vi "Create.vi"(8 "error in (no error)":errorcluster, 10 "Debug Data Cluster":T1) -> (0 "error out":errorcluster, 3 "Debug Data out":refnum<class "Debug Data.lvclass">)   [LabVIEW 2020, in "Debug Data.lvclass"]
uses:
  Debug Data.lvclass
  Raw Debug Data.ctl
  Debug Data.lvclass/Debug Data.ctl
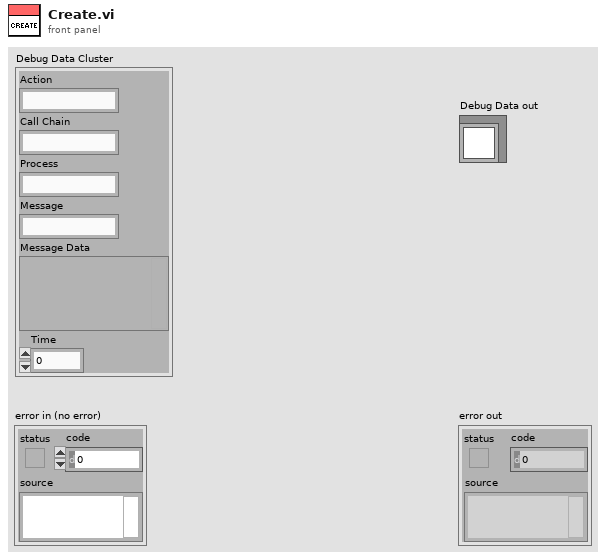
[diagram p1: front panel]
types:
  T1 = typedef "Debug Data.lvclass/Raw Debug Data.ctl" = cluster{"Action":string, "Call Chain":string, "Process":string, "Message":string, "Message Data":variant, "Time":dbl}
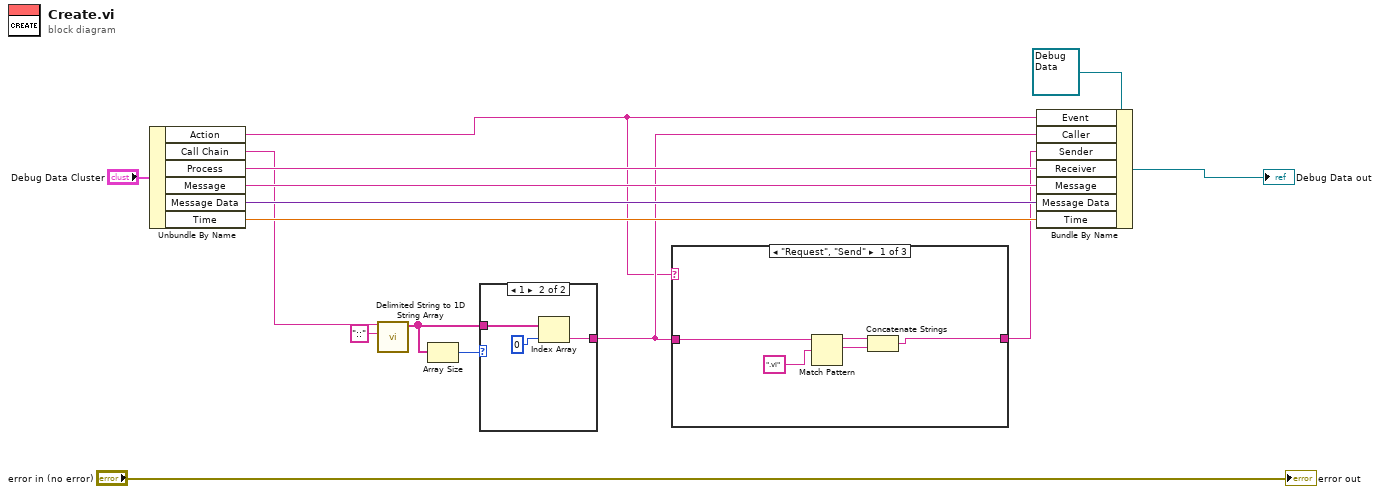
[diagram p0: block diagram]
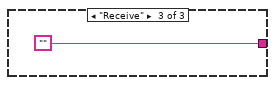
[diagram p3: hidden frame]
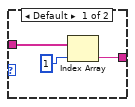
[diagram p4: hidden frame]
diagram:
  n1 = Unbundle By Name("Debug Data Cluster") -> ("Action"=w1:string, "Call Chain"=w4:string, "Process"=w12:string, "Message"=w11:string, "Message Data"=w10:variant, "Time"=w9:dbl)
  n2 = call <vilib>:"Delimited String to 1D String Array.vi"("delimiter"="::", "delimited string"=w4) -> ("string array"=w6:string[])  [unwired: 9 in]
  n3 = Array Size(array=w6) -> (size(s)=w5:i32)
  n4 = case shown="1" w5 {
    tunnel: [w18 w21] -> w3
    tunnel: w6 -> [w16 w19]
    frame Default {
      n5 = Index Array(array=w16, index=1) -> (element=w18:string)
    }
    frame 1 {
      n6 = Index Array(array=w19, index=0) -> (element=w21:string)
    }
  }
  n7 = case shown="\"Request\", \"Send\"" w1 {
    tunnel: w3 -> [w25 w27 _]
    tunnel: [w22 w27 "" ("String")] -> w2
    frame "Request", "Send" {
      n8 = Match Pattern(string=w25, regular expression=".vi") -> (before substring=w24:string, match substring=w23:string)  [unwired: 1 in, 2 out]
      n9 = Concatenate Strings(w24, w23) -> (w22:string)
    }
    frame Default {
    }
    frame "Receive" {
    }
  }
  n10 = Bundle By Name(cluster=refnum<class "Debug Data.lvclass"> refnum ("Debug Data out"), "Event"=w1, "Caller"=w3, "Sender"=w2, "Receiver"=w12, "Message"=w11, "Message Data"=w10, "Time"=w9) -> (→"Debug Data out":refnum<class "Debug Data.lvclass">)
  "error out" <- "error in (no error)"
